vi "getDeviceType.vi"(8 "error in":errorcluster, 10 "Device Type in":string, 11 "connection ID":refnum<k5>) -> (0 "error out":errorcluster, 2 "Device Type out":string, 3 "connection ID":refnum<k5>)   [LabVIEW 2019]
panel:
  in  "Get Command":string="com.attocube.amc.description.getDeviceType"
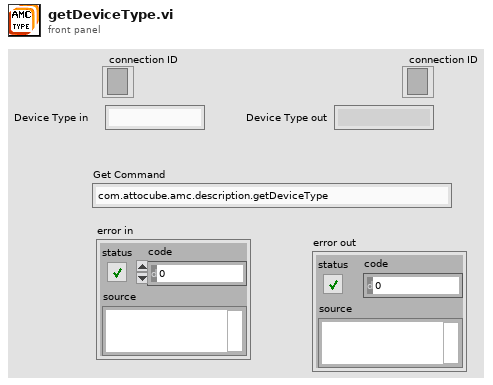
[diagram p1: front panel]
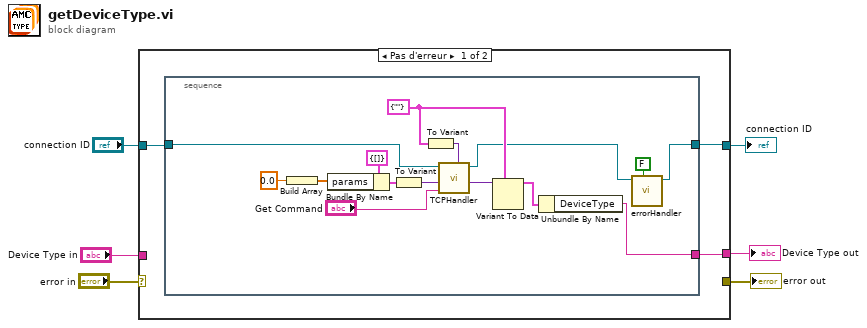
[diagram p0: block diagram]
diagram:
  n1 = case shown="Pas d'erreur" "error in" {
    selector: "error in" -> [_ w26]
    tunnel: [_ w26] -> w6
    tunnel: "Device Type in" -> [_ w27]
    tunnel: [w8 w27] -> w4
    tunnel: [w7 w25] -> w3
    tunnel: "connection ID" -> [w9 w25]
    frame No Error {
      n2 = stacked-sequence {
        tunnel: [w10] -> w7
        tunnel: w9 -> [w17]
        tunnel: [w14] -> w8
        frame #0 {
          w15 = cluster{"DeviceType":string} {"DeviceType"=""} ("input cluster")
          n3 = Build Array(0.0 ("element")) -> (w21:dbl[])
          n4 = Bundle By Name(cluster=cluster{"params":i16[]} {"params"=[]} ("input cluster"), "params"=w21) -> (w22:cluster{"params":i16[]})
          n5 = To Variant(anything=w22) -> (Variant=w23:variant)
          n6 = To Variant(anything=w15) -> (Variant=w16:variant)
          n7 = call "TCPHandler.vi"("result Types"=w16, "method"="Get Command", "params"=w23, "connection ID"=w17) -> ("result"=w19:variant, "connection ID"=w11:refnum<k5>)  [unwired: 5 in, 1 out]
          n8 = Variant To Data(type=w15, Variant=w19) -> (data=w24:cluster{"DeviceType":string})  [unwired: 1 in, 1 out]
          n9 = Unbundle By Name(w24) -> ("DeviceType"=w14:string)
          n10 = call "errorHandler.vi"("show popup"=FALSE, "connection ID"=w11) -> ("connection ID"=w10:refnum<k5>)  [unwired: 8 in, 1 out]
        }
      }
    }
    frame Error {
    }
  }
  "error out" <- w6
  "Device Type out" <- w4
  "connection ID" <- w3
